vi "LabView_Test.vi"() -> ()   [LabVIEW 2018]
panel:
  in  "숫자형 6":dbl
  out "y":dbl
  out "숫자형 4":dbl
  out "슬라이드":dbl(slide) scale=0.0..100.0 scale format="%#_10g"
  in  "숫자형 3":dbl
  in  "숫자형 2":dbl
  in  "숫자형":dbl
  in  "노브":dbl(knob) scale=0.0..10.0
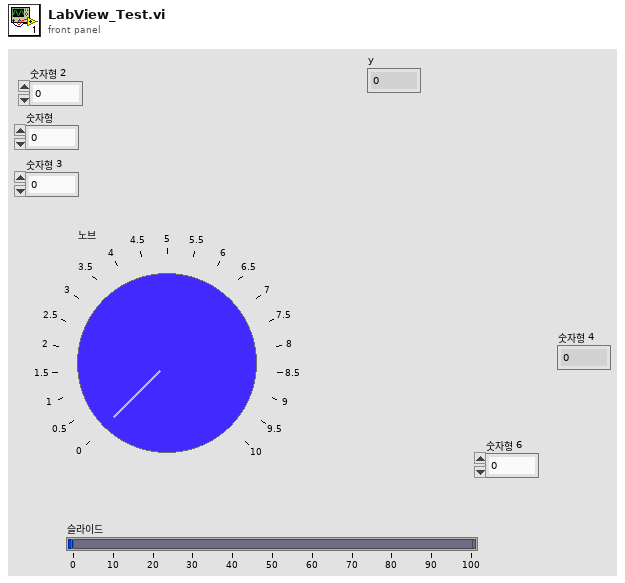
[diagram p1: front panel]
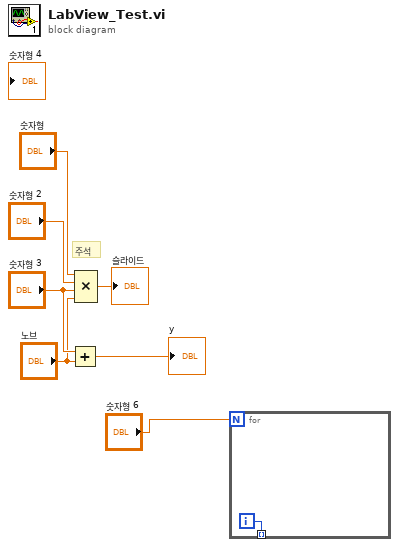
[diagram p0: block diagram]
diagram:
  # "주석"
  n1 = Add(x="숫자형 3", y="노브") -> (x+y=→"y":dbl)
  n2 = Compound Arithmetic op=MULTIPLY ("복합 연산")("숫자형", "숫자형 2", "숫자형 3", "노브") -> (→"슬라이드":dbl)
  n3 = for {
    N: "숫자형 6" -> [_]
    tunnel: [w8] -> _ mode=indexing
    i -> [w8]
  }
